vi "json Parse Float Array - array path.vi"(6 "use default?":bool=TRUE, 8 "error in (no error)":errorcluster, 9 "default":sgl[](array[numeric]), 10 "path":string[](array[string]), 11 "JSON Document in":refnum<class "JSON Document.lvclass">) -> (0 "error out":errorcluster, 1 "defaulted?":bool, 2 "value":sgl[](array[numeric]), 3 "JSON Document out":refnum<class "JSON Document.lvclass">, 4 "elements defaulted?":bool[](array[boolean]))   [LabVIEW 2015, in "JSON Document.lvclass"]
uses:
  JSON Document.lvclass
  json Parse Float Array - string path.vi
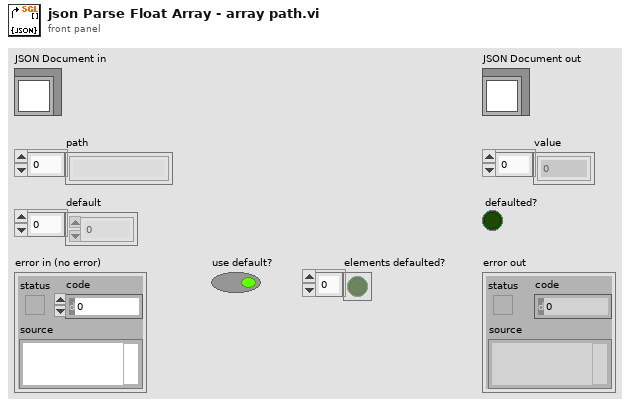
[diagram p1: front panel]
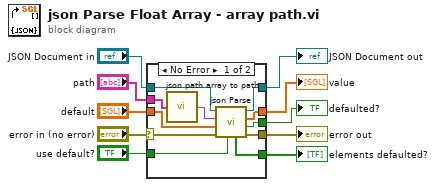
[diagram p0: block diagram]
diagram:
  n1 = case shown="No Error" "error in (no error)" {
    selector: "error in (no error)" -> [w16 w24]
    tunnel: [w17 w24] -> w9
    tunnel: [w20 w23] -> w7
    tunnel: "JSON Document in" -> [w21 w23]
    tunnel: "default" -> [w14 w22]
    tunnel: "path" -> [w15 _]
    tunnel: [w18 w22] -> w4
    tunnel: [w19 _] -> w3
    tunnel: [w13 _] -> w2
    tunnel: "use default?" -> [w11 _]
    frame No Error {
      n2 = call "json path array to path.vi"("path"=w15) -> ("String"=w12:string)
      n3 = call-poly "json Parse.vi"("use default?"=w11, "error in (no error)"=w16, "default"=w14, "path"=w12, "JSON Document in"=w21) -> ("error out"=w17:errorcluster, "defaulted?"=w19:bool, "value"=w18:sgl[], "JSON Document out"=w20:refnum<class "JSON Document.lvclass">, "elements defaulted?"=w13:bool[])  [unwired: 2 in]
    }
    frame Error {
    }
  }
  "error out" <- w9
  "JSON Document out" <- w7
  "value" <- w4
  "defaulted?" <- w3
  "elements defaulted?" <- w2
